vi "power out.vi"(7 "Max Voltage in (V)":dbl=8.5 format="%.2f", 9 "Normalized Power (0-1)":dbl format="%.2f", 11 "error in (no error)":errorcluster) -> (8 "Max Voltage out (V)":dbl=8.5 format="%.2f", 15 "error out":errorcluster)   [LabVIEW 2014]
doc: "This one shot VI sets the power out via analog out. The output can be cleared by running the vi again with the Clear button set to true. If this fails power off the NI Elvis Board.\n\nMatt Strader\nPaul K Dixon\nPhysics 350\nCSUSB Physics"
panel:
  in  "Clear":bool
  in  "Device":tag="Dev1"
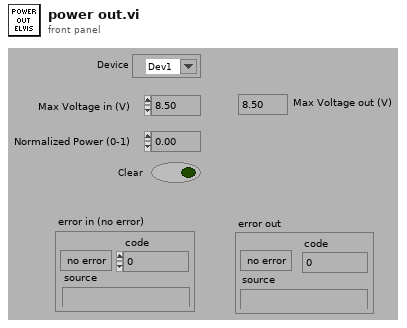
[diagram p1: front panel]
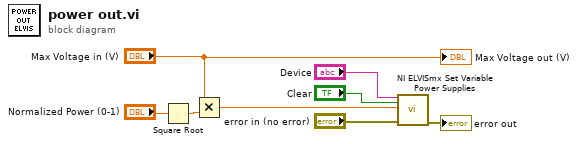
[diagram p0: block diagram]
diagram:
  n1 = Square Root(x="Normalized Power (0-1)") -> (sqrt(x)=w7:dbl)
  n2 = Multiply(x="Max Voltage in (V)", y=w7) -> (x*y=w3:dbl)
  n3 = call "NI ELVISmx Set Variable Power Supplies.vi"("Device Name"="Device", "Stop"="Clear", "Supply+ (V)"=w3, "error in"="error in (no error)") -> ("error out"=→"error out":errorcluster)  [unwired: 3 in, 12 out]
  "Max Voltage out (V)" <- "Max Voltage in (V)"
